vi "SetLvLibPath.vi"(0 "LibWriter":refnum<class "LibWriter.lvclass">, 1 "LibPath":path, 2 "LibName":string, 5 "error in (no error)":errorcluster) -> (14 "LibWriter":refnum<class "LibWriter.lvclass">, 19 "error out":errorcluster)   [LabVIEW 2014, in "LibWriter.lvclass"]
uses:
  <resource>/Framework/Providers/Open_GDS/ClassProviders/LibProvider_BaseClassInterface/LibWriter_class/ClassWriter_class/LibWriter.lvclass
  <resource>/Framework/Providers/Open_GDS/ClassProviders/LibProvider_BaseClassInterface/LibWriter_class/ClassWriter_class/LibWriter.lvclass/LibWriter.ctl
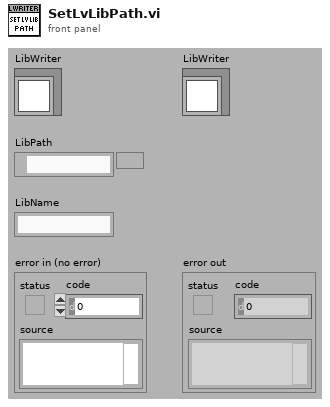
[diagram p1: front panel]
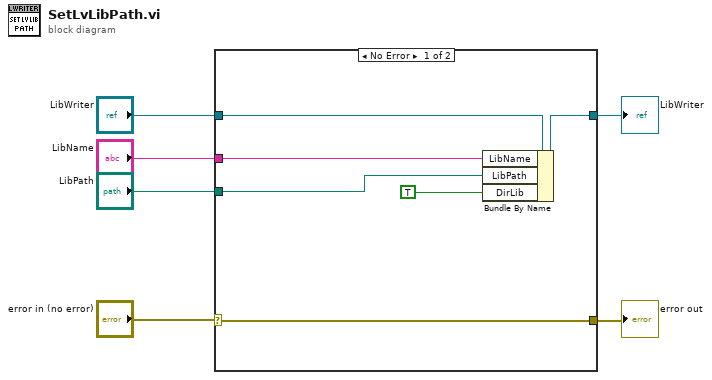
[diagram p0: block diagram]
diagram:
  n1 = case shown="No Error" "error in (no error)" {
    selector: "error in (no error)" -> [w10 w13]
    tunnel: "LibWriter" -> [w12 w14]
    tunnel: [w11 w14] -> w5
    tunnel: [w10 w13] -> w3
    tunnel: "LibPath" -> [w9 _]
    tunnel: "LibName" -> [w7 _]
    frame No Error {
      n2 = Bundle By Name(cluster=w12, "LibName"=w7, "LibPath"=w9, "DirLib"=TRUE ("DirClass")) -> (w11:refnum<class "LibWriter.lvclass">)
    }
    frame Error {
    }
  }
  "LibWriter" <- w5
  "error out" <- w3
